vi "Configure Output Delay.vi"(7 "Disabled Output Delay (0.0 s)":dbl format="%^.3e", 8 "error in (no error)":errorcluster {"code" format="%.0x"}, 9 "Enabled Output Delay (0.0 s)":dbl format="%^.3e", 10 "Channel Name (1)":string="1", 11 "VISA resource name":refnum<visa-resource-name>) -> (0 "error out":errorcluster {"code" format="%.0x"}, 3 "VISA resource name out":refnum<visa-resource-name>)   [LabVIEW 2014, in "Agilent N6700 Series.lvlib"]
doc: "Sets the delay in seconds that the instrument waits before enabling and disabling the specified channel output."
uses:
  Agilent N6700 Series.lvlib
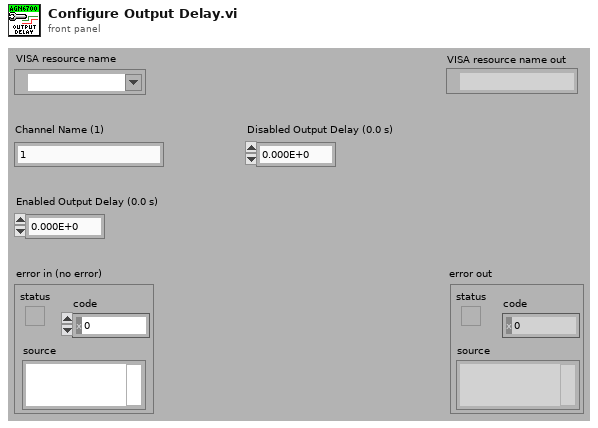
[diagram p1: front panel]
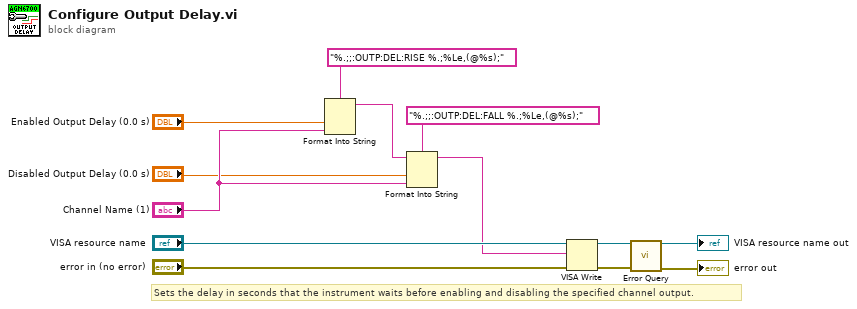
[diagram p0: block diagram]
diagram:
  # "Sets the delay in seconds that the instrument waits before enabling and disabling the specified channel output."
  n1 = Format Into String(format string="%.;;:OUTP:DEL:RISE %.;%Le,(@%s);", "Enabled Output Delay (0.0 s)", "Channel Name (1)") -> (resulting string=w7:string)  [unwired: 2 in, 1 out]
  n2 = Format Into String(format string="%.;;:OUTP:DEL:FALL %.;%Le,(@%s);", initial string=w7, "Disabled Output Delay (0.0 s)", "Channel Name (1)") -> (resulting string=w6:string)  [unwired: 1 in, 1 out]
  n3 = VISA Write(VISA resource name="VISA resource name", write buffer=w6, error in (no error)="error in (no error)") -> (VISA resource name out=w9:refnum<visa-resource-name>, error out=w8:errorcluster)  [unwired: 1 out]
  n4 = call "Error Query.vi"("VISA resource name"=w9, "error in (no error)"=w8) -> ("VISA resource name out"=→"VISA resource name out":refnum<visa-resource-name>, "error out"=→"error out":errorcluster)  [unwired: 10 in, 2 out]
